vi "Execute.vi"(8 "error in (no error)":errorcluster, 9 "Consumer Queues in":T1, 10 "DAC Process Command in":refnum<class "Configure DAC Front Panel.lvclass">, 11 "DAC Process Data in":T2) -> (0 "error out":errorcluster, 1 "Consumer Queues out":T1, 2 "Stop?":bool, 3 "DAC Process Data out":T2)   [LabVIEW 2019, in "DAC Process.lvlib" / "Configure DAC Front Panel.lvclass"]
uses:
  Configure DAC Front Panel.lvclass
  DAC Process Data.ctl
  Generic Test Stand/Generic Test Stand.lvclass
  TS Framework/ExeLogging/DAC Logger/DAC Logger.lvclass
  DAC State.ctl
  TS Framework/Consumer Queues.ctl
  UI Process/Generic UI Command/Generic UI Process Command.lvclass
  Generic DAC Command/Generic DAC Process Command.lvclass
  Trig Process/Generic Trig Command/Generic Trig Process Command.lvclass
  Run DAC Front Panel/Run DAC Front Panel.lvclass
  Run DAC Front Panel/Run DAC Front Panel.lvclass/Run DAC Front Panel.ctl
  DAC Process.lvlib
  TS Framework/TS Framework.lvlib
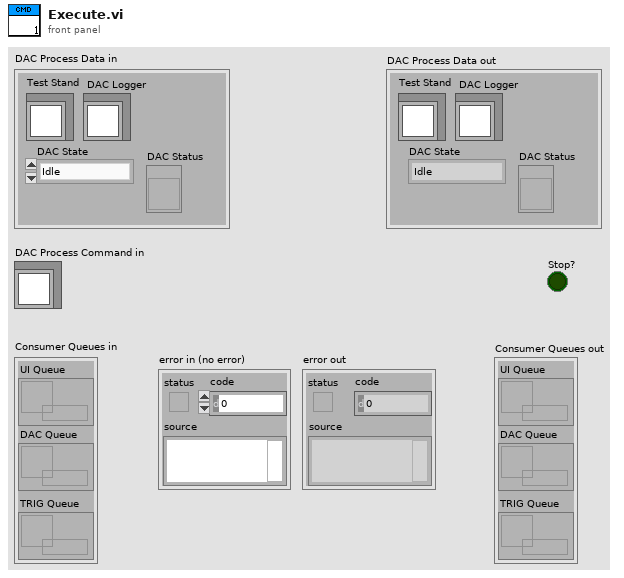
[diagram p1: front panel]
types:
  T1 = typedef "TS Framework.lvlib/Consumer Queues.ctl" = cluster{"UI Queue":refnum<queue>, "DAC Queue":refnum<queue>, "TRIG Queue":refnum<queue>}
  T2 = typedef "DAC Process.lvlib/DAC Process Data.ctl" = cluster{"Test Stand":refnum<class "Generic Test Stand.lvclass">, " DAC Logger":refnum<class "DAC Logger.lvclass">, "DAC State":T3, "DAC Status":refnum<vi>}
  T3 = typedef "DAC Process.lvlib/DAC State.ctl" = enum16{"Idle", "Acquiring"}
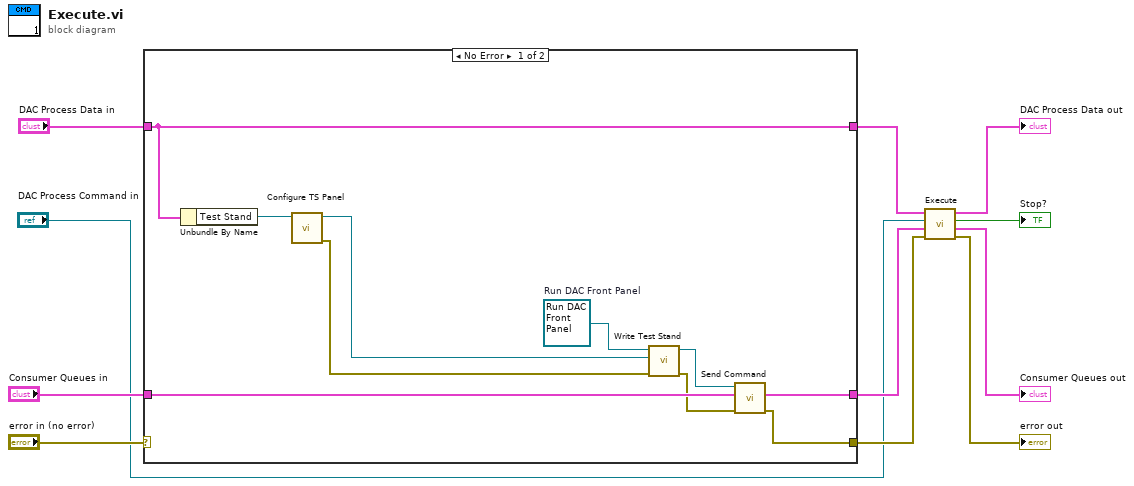
[diagram p0: block diagram]
diagram:
  n1 = case shown="No Error" "error in (no error)" {
    selector: "error in (no error)" -> [_ w22]
    tunnel: "Consumer Queues in" -> [w21 w23]
    tunnel: "DAC Process Data in" -> [w17 w24]
    tunnel: [w17 w24] -> w4
    tunnel: [w15 w22] -> w3
    tunnel: [w20 w23] -> w2
    frame No Error {
      w19 = refnum<class "Run DAC Front Panel.lvclass"> refnum  # Run DAC Front Panel
      n2 = Unbundle By Name(w17) -> ("Test Stand"=w13:refnum<class "Generic Test Stand.lvclass">)
      n3 = call-dynamic "Configure TS Panel.vi"("Generic Test Stand in"=w13) -> ("error out"=w12:errorcluster, "Generic Test Stand out"=w14:refnum<class "Generic Test Stand.lvclass">)  [unwired: 9 in]
      n4 = call "Write Test Stand.vi"("error in (no error)"=w12, "Generic Test Stand.lvclass"=w14, "Run DAC Front Panel in"=w19) -> ("error out"=w16:errorcluster, "Run DAC Front Panel out"=w18:refnum<class "Run DAC Front Panel.lvclass">)  [unwired: 7 in]
      n5 = call-dynamic "Send Command.vi"("error in (no error)"=w16, "Consumer Queues in"=w21, "DAC Process Command"=w18) -> ("error out"=w15:errorcluster, "Consumer Queues out"=w20:T1)  [unwired: 7 in]
    }
    frame Error {
    }
  }
  n6 = call-parent "Execute.vi"("error in"=w3, "Consumer Queues in"=w2, "DAC Process Command in"="DAC Process Command in", "DAC Process Data in"=w4) -> ("error out"=→"error out":errorcluster, "Consumer Queues out"=→"Consumer Queues out":T1, "Stop?"=→"Stop?":bool, "DAC Process Data out"=→"DAC Process Data out":T2)  [unwired: 4 in]
